vi "MPM_Set_Sweep_Wavelength.vi"(7 "wavestep":dbl, 8 "error in (no error)":errorcluster, 9 "stopwave":dbl, 10 "startwave":dbl, 11 ".NET Reference in":refnum<k24>) -> (0 "error out":errorcluster, 3 "Reference out":refnum<k24>)   [LabVIEW 2017]
uses:
  LV_IL_Sample/DLL/InstrumentDLL.dll
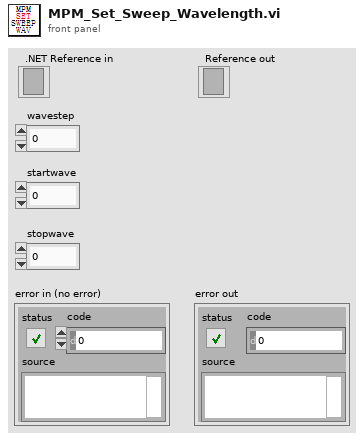
[diagram p1: front panel]
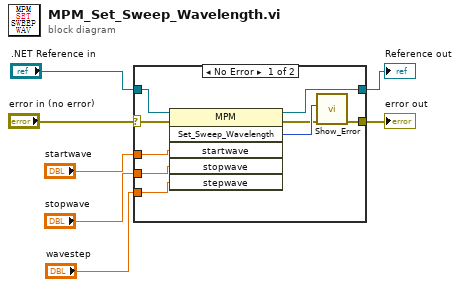
[diagram p0: block diagram]
diagram:
  n1 = case shown="No Error" "error in (no error)" {
    selector: "error in (no error)" -> [w10 w18]
    tunnel: "wavestep" -> [w16 _]
    tunnel: "stopwave" -> [w15 _]
    tunnel: "startwave" -> [w14 _]
    tunnel: [w11 w18] -> w4
    tunnel: ".NET Reference in" -> [w9 w17]
    tunnel: [w8 w17] -> w1
    frame No Error {
      n2 = invoke class="MPM" method="Set_Sweep_Wavelength"(reference=w9, error in=w10, "startwave"=w14, "stopwave"=w15, "stepwave"=w16) -> (reference out=w8:refnum<k24>, error out=w12:errorcluster, "Set_Sweep_Wavelength"=w13:i32)  [unwired: 1 in, 3 out]
      n3 = call "Show_Error.vi"("error in (no error)"=w12, "Error"=w13) -> ("error out"=w11:errorcluster)  [unwired: 9 in]
    }
    frame Error {
    }
  }
  "Reference out" <- w1
  "error out" <- w4
